vi "Change the Theme.vi"() -> ()   [LabVIEW 2021]
uses:
  Material Theme/Material Theme.lvclass
panel:
  out "error out":errorcluster
  in  "Theme":u16(ring)=3 items=["Light Theme", "Light Medium Contrast", "Light High Contrast", "Dark Theme", "Dark Medium Contrast", "Dark High Constrast"]
  in  "file path (use dialog)":path
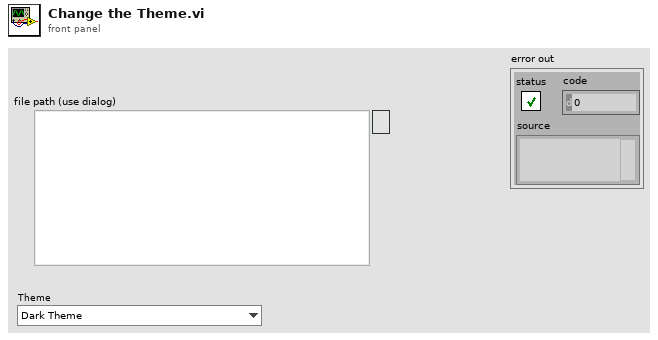
[diagram p1: front panel]
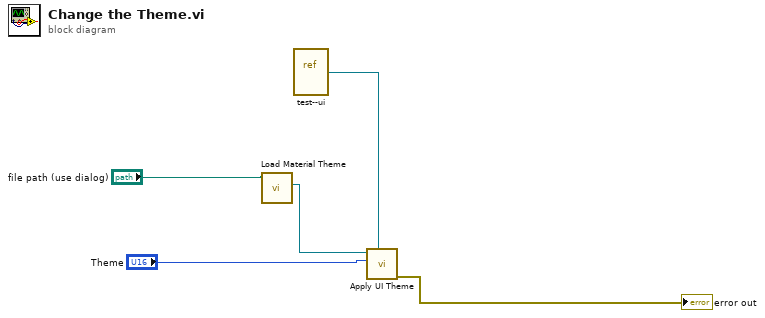
[diagram p0: block diagram]
diagram:
  n1 = call "Load Material Theme.vi"("file path (use dialog)"="file path (use dialog)") -> ("Theme"=w4:refnum<class "Material Theme.lvclass">)  [unwired: 9 in, 1 out]
  n2 = vi-ref "test--ui.vi"() -> (w2:refnum<vi>)
  n3 = call "Apply UI Theme.vi"("VI Refnum"=w2, "Theme"="Theme", "Material Theme in"=w4) -> ("error out"=→"error out":errorcluster)  [unwired: 7 in, 1 out]
